vi "Set Address Globalvi.vi"() -> ()   [LabVIEW 2009]
uses:
  Utility VI's/Message VI's/Message Address Global.vi
panel:
  in  "Boolean":bool
  in  "Option 2":T1(array[cluster])=[{"Module"="QCA", "Address"="132.177.89.194", "Port"=9326}, {"Module"="PDP", "Address"="132.177.89.194", "Port"=9327}, {"Module"="TEB", "Address"="132.177.89.194", "Port"=9328}, {"Module"="TCL", "Address"="132.177.89.194", "Port"=9329}, {"Module"="OLA", "Address"="132.177.89.194", "Port"=9330}, {"Module"="SMC", "Address"="132.177.89.194", "Port"=9331}]
  in  "Option 1":T1(array[cluster])=[{"Module"="QCA", "Address"="132.177.89.194", "Port"=9326}, {"Module"="PDP", "Address"="132.177.89.194", "Port"=9327}, {"Module"="TEB", "Address"="132.177.89.194", "Port"=9328}, {"Module"="TCL", "Address"="132.177.89.194", "Port"=9329}, {"Module"="OLA", "Address"="132.177.89.194", "Port"=9330}, {"Module"="SMC", "Address"="132.177.89.194", "Port"=9331}]
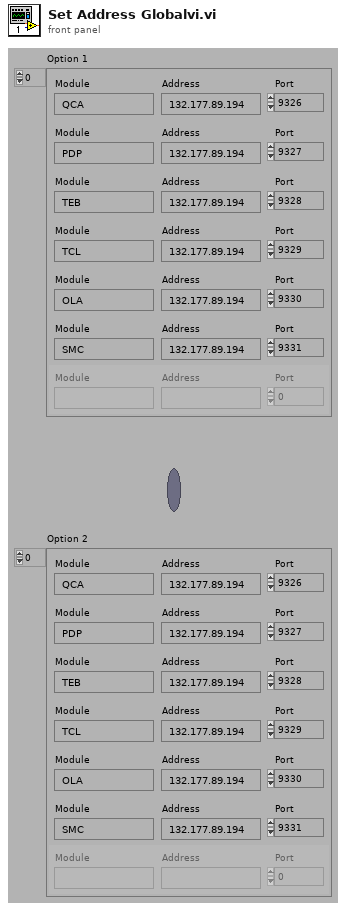
[diagram p1: front panel]
types:
  T1 = cluster{"Module":string, "Address":string, "Port":u16}[]
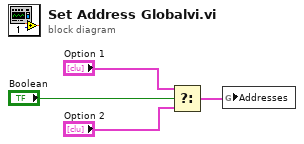
[diagram p0: block diagram]
diagram:
  n1 = Select(t="Option 1", s="Boolean", f="Option 2") -> (s? t:f=w4:T1)
  n2 = global write "Message Address Global.vi" "Addresses"(w4) -> ()
